vi "gather_compass_data.vi"(10 "data in":T1, 11 "VISA Refnum in":refnum<visa-resource-name>) -> (1 "next timeout (ms)":i32, 2 "data out":T1, 3 "VISA Refnum out":refnum<visa-resource-name>)   [LabVIEW 2019, in "Nano33BLE-TiltCompensationSupport.lvlib"]
uses:
  types/compass_data.ctl
  types/xyz.ctl
  Nano33BLE-TiltCompensationSupport.lvlib
  <vilib>/ptbypt/NI_PtbyPt.lvlib
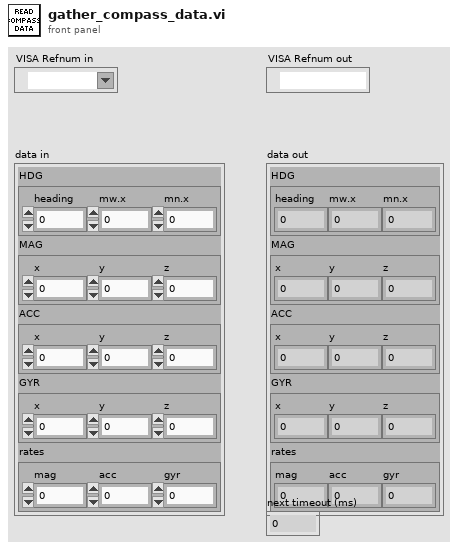
[diagram p1: front panel]
types:
  T1 = typedef "Nano33BLE-TiltCompensationSupport.lvlib/compass_data.ctl" = cluster{"HDG":cluster{"heading":dbl, "mw.x":dbl, "mn.x":dbl}, "MAG":T2, "ACC":T2, "GYR":T2, "rates":cluster{"mag":dbl, "acc":dbl, "gyr":dbl}}
  T2 = typedef "Nano33BLE-TiltCompensationSupport.lvlib/xyz.ctl" = cluster{"x":dbl, "y":dbl, "z":dbl}
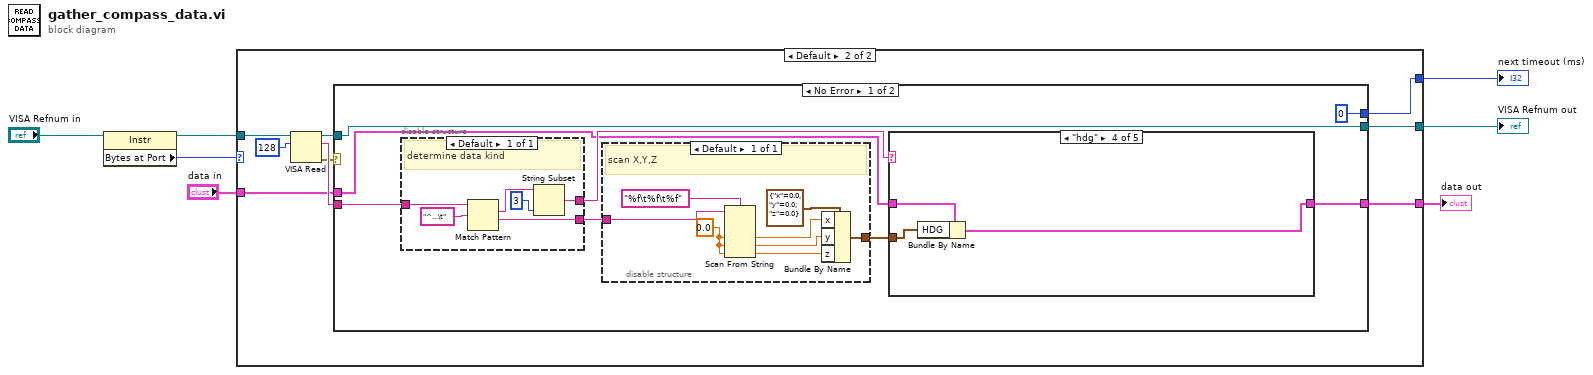
[diagram p0: block diagram]
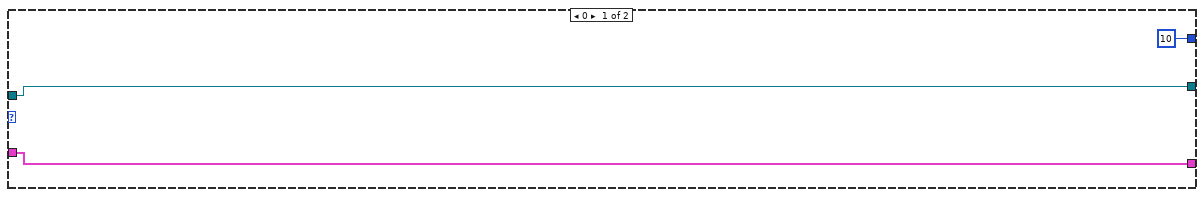
[diagram p2: hidden frame]
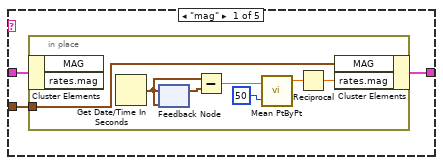
[diagram p3: hidden frame]
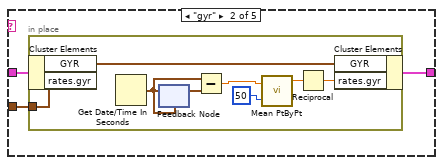
[diagram p4: hidden frame]
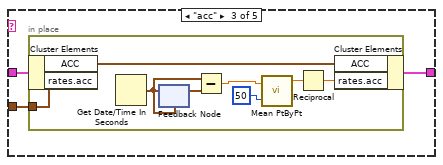
[diagram p5: hidden frame]
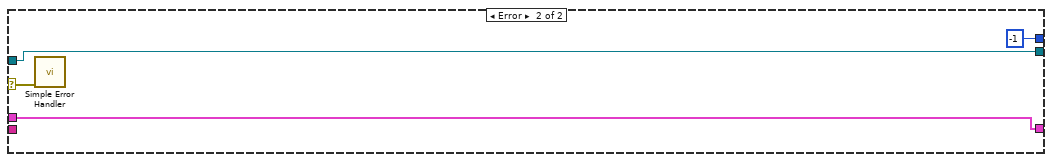
[diagram p7: hidden frame]
diagram:
  n1 = property class="Instr"(reference="VISA Refnum in") -> (reference out=w5:refnum<visa-resource-name>, "Bytes at Port"=w4:u32)  [unwired: 1 in, 1 out]
  n2 = case shown="Default" w4 {
    tunnel: w5 -> [w9 w17]
    tunnel: [10 w13] -> w6
    tunnel: [w9 w14] -> w7
    tunnel: [w8 w12] -> w1
    tunnel: "data in" -> [w8 w11]
    frame 0 {
    }
    frame Default {
      n3 = VISA Read(VISA resource name=w17, byte count=u32 128) -> (VISA resource name out=w15:refnum<visa-resource-name>, read buffer=w18:string, error out=w16:errorcluster)  [unwired: 1 in, 1 out]
      n4 = case shown="No Error" w16 {
        selector: w16 -> [_ w79]
        tunnel: w18 -> [w27 _]
        tunnel: w15 -> [w25 w78]
        tunnel: [w25 w78] -> w14
        tunnel: [0 -1] -> w13
        tunnel: [w23 w76] -> w12
        tunnel: w11 -> [w20 w76]
        frame No Error {
          n5 = disable-structure shown="Default" {
            disable-tunnel: w27 -> [w32]
            disable-tunnel: [w29] -> w26
            disable-tunnel: [w28] -> w22
            frame Enabled {
              # "determine data kind"
              n6 = Match Pattern(string=w32, regular expression="^...\t") -> (match substring=w30:string, after substring=w28:string)  [unwired: 1 in, 2 out]
              n7 = String Subset(string=w30, length (rest)=3 ("length (rest)")) -> (substring=w29:string)  [unwired: 1 in]
            }
          }
          n8 = disable-structure shown="Default" {
            disable-tunnel: w22 -> [w39]
            disable-tunnel: [w34] -> w21
            frame Enabled {
              w40 = 0.0 ("default value 1")
              # "scan X,Y,Z"
              n9 = Scan From String(format string="%f\t%f\t%f", input string=w39, default 1=w40, default 2=w40, default 3=w40) -> (output 1=w38:dbl, output 2=w37:dbl, output 3=w36:dbl)  [unwired: 2 in, 3 out]
              n10 = Bundle By Name(cluster=T2 {"x"=0.0, "y"=0.0, "z"=0.0} ("xyz"), "x"=w38, "y"=w37, "z"=w36) -> (w34:T2)
            }
          }
          n11 = case shown="\"hdg\"" w26 {
            tunnel: [w43 w52 w62 w73 w75] -> w23
            tunnel: w21 -> [w44 w54 w64 w72 _]
            tunnel: w20 -> [w42 w53 w63 w74 w75]
            frame "mag" {
              n12 = in-place {
                in-place-border: w44 -> [w45]
                n13 = in-place-cluster #1(w42) -> ()  [unwired: 2 out]
                n14 = Get Date/Time In Seconds() -> (seconds since 1Jan1904=w46:timestamp)
                n15 = feedback-in #2(w46) -> ()
                n16 = feedback #2(w46) -> (w51:timestamp)
                n17 = Subtract(x=w46, y=w51) -> (x-y=w50:dbl)
                n18 = call <vilib>:"Mean PtByPt.vi"("x"=w50, "sample length"=50) -> ("mean"=w48:dbl)  [unwired: 2 in, 1 out]
                n19 = Reciprocal(x=w48) -> (1/x=w47:dbl)
                n20 = in-place-cluster #1("MAG"=w45, "rates.mag"=w47) -> (w43:T1)
              }
            }
            frame "gyr" {
              n21 = in-place {
                in-place-border: w54 -> [w55]
                n22 = in-place-cluster #3(w53) -> ()  [unwired: 2 out]
                n23 = Get Date/Time In Seconds() -> (seconds since 1Jan1904=w56:timestamp)
                n24 = feedback #4(w56) -> (w61:timestamp)
                n25 = feedback-in #4(w56) -> ()
                n26 = Subtract(x=w56, y=w61) -> (x-y=w60:dbl)
                n27 = call <vilib>:"Mean PtByPt.vi"("x"=w60, "sample length"=50) -> ("mean"=w59:dbl)  [unwired: 2 in, 1 out]
                n28 = Reciprocal(x=w59) -> (1/x=w57:dbl)
                n29 = in-place-cluster #3("GYR"=w55, "rates.gyr"=w57) -> (w52:T1)
              }
            }
            frame "acc" {
              n30 = in-place {
                in-place-border: w64 -> [w65]
                n31 = in-place-cluster #5(w63) -> ()  [unwired: 2 out]
                n32 = Get Date/Time In Seconds() -> (seconds since 1Jan1904=w66:timestamp)
                n33 = feedback #6(w66) -> (w71:timestamp)
                n34 = feedback-in #6(w66) -> ()
                n35 = Subtract(x=w66, y=w71) -> (x-y=w70:dbl)
                n36 = call <vilib>:"Mean PtByPt.vi"("x"=w70, "sample length"=50) -> ("mean"=w69:dbl)  [unwired: 2 in, 1 out]
                n37 = Reciprocal(x=w69) -> (1/x=w67:dbl)
                n38 = in-place-cluster #5("ACC"=w65, "rates.acc"=w67) -> (w62:T1)
              }
            }
            frame "hdg" {
              n39 = Bundle By Name(cluster=w74, "HDG"=w72) -> (w73:T1)
            }
            frame Default {
            }
          }
        }
        frame Error {
          n40 = call <vilib>:"Simple Error Handler.vi"("error in (no error)"=w79) -> ()  [unwired: 4 in, 5 out]
        }
      }
    }
  }
  "data out" <- w1
  "VISA Refnum out" <- w7
  "next timeout (ms)" <- w6
